vi "Close.vi"(8 "error in (no error)":errorcluster, 11 "Ethernet in":refnum<class "TCP.lvclass">) -> (0 "error out":errorcluster, 3 "Ethernet out":refnum<class "TCP.lvclass">)   [LabVIEW 2023, in "Protocols.lvlib" / "TCP.lvclass"]
uses:
  TCP.lvclass
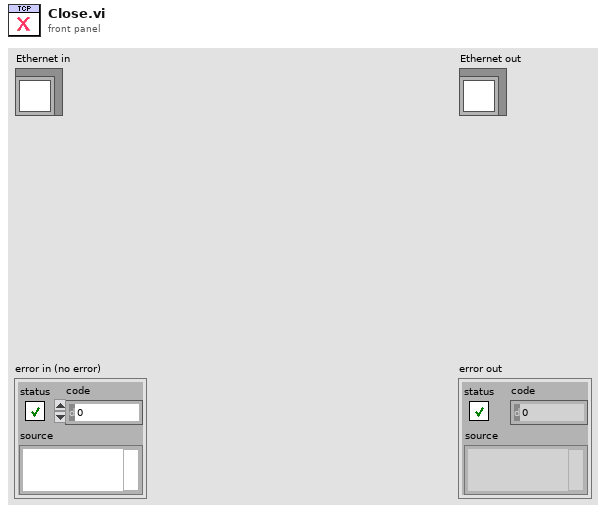
[diagram p1: front panel]
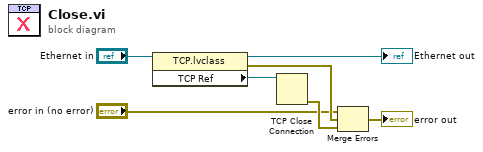
[diagram p0: block diagram]
diagram:
  n1 = property class="TCP.lvclass"(reference="Ethernet in") -> (reference out=→"Ethernet out":refnum<class "TCP.lvclass">, error out=w5:errorcluster, "TCP Ref"=w7:refnum<k5>)  [unwired: 1 in]
  n2 = TCP Close Connection(connection ID=w7) -> (error out=w6:errorcluster)  [unwired: 2 in, 1 out]
  n3 = Merge Errors("error in (no error)", w5, w6) -> (→"error out":errorcluster)
